vi "CalculateZ.vi"(5 "File Path to Save":path, 7 "EIS File":bool, 8 "Avg I & V":waveform(dbl)[](graph) caption="I & V WFM", 11 "Frequency":dbl format="%.6f") -> (0 "Nyquist Plot":cluster{"Y":dbl[], "Y":dbl[]}[](graph), 1 "ZIm":dbl, 2 "ZRe":dbl, 3 "Current Frequency":dbl format="%.2p", 4 "Ztheta":dbl, 6 "ZMag":dbl)   [LabVIEW 2018]
uses:
  <vilib>/measure/matone.llb/Extract Single Tone Information 1 Chan.vi
  <vilib>/Utility/file.llb/Write To Spreadsheet File (DBL).vi
  <vilib>/measure/NI_MAPro.lvlib
panel:
  out "Avg Voltage":waveform(dbl)(graph)
  out "Avg Current":waveform(dbl)(graph)
  out "Voltage Phase (deg)":dbl format="%.2p"
  out "Voltage Amplitude (V)":dbl format="%.2p"
  out "Voltage Frequency":dbl format="%.2p"
  out "Current Phase (deg)":dbl format="%.2p"
  out "Current Amplitude (A)":dbl format="%.2p"
  # "Inputs"
  # "Outputs"
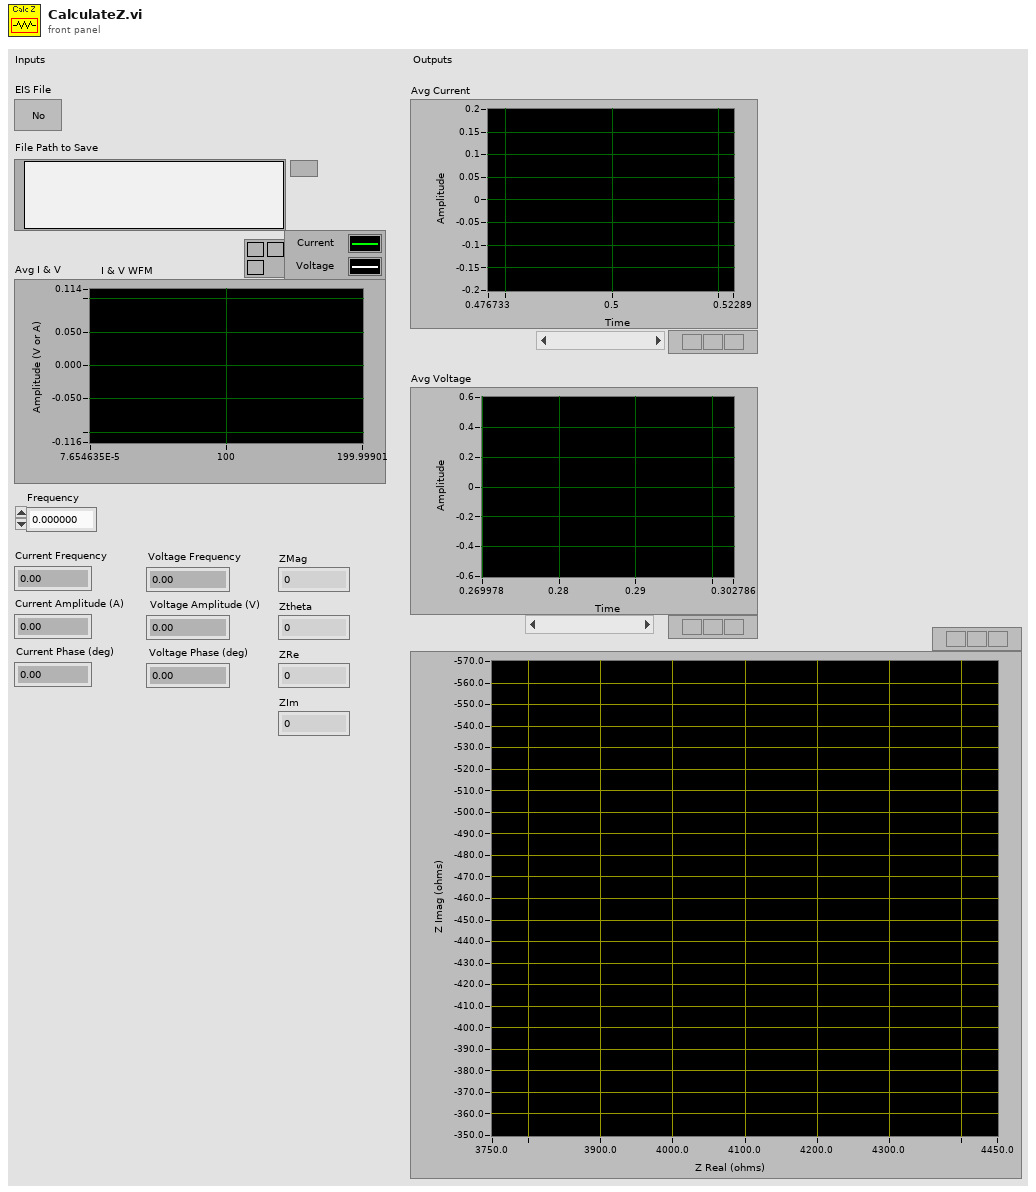
[diagram p1: front panel]
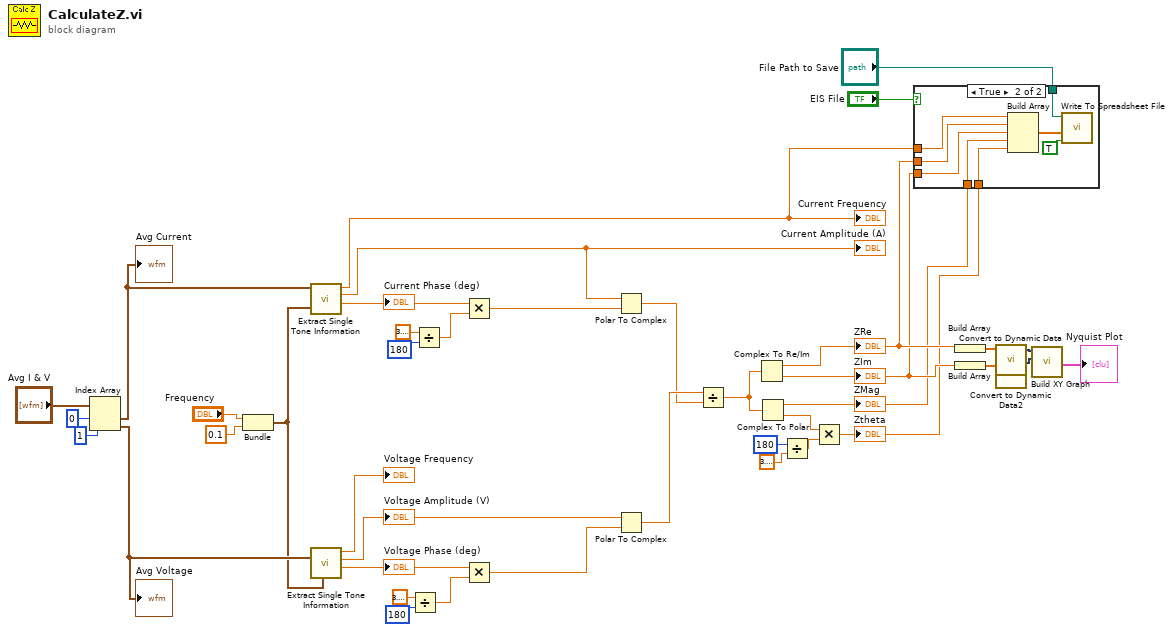
[diagram p0: block diagram]
diagram:
  n1 = Index Array(array="Avg I & V", index #1=0 ("index"), index #2=1 ("index")) -> (element #1=w16:waveform(dbl), element #2=w15:waveform(dbl))
  "Avg Current" <- w16
  "Avg Voltage" <- w15
  n2 = Bundle("Frequency"="Frequency", 0.1) -> (w13:cluster{"Frequency":dbl, dbl})  [unwired: 1 in]
  n3 = call-poly <vilib>:"Extract Single Tone Information.vi"("advanced search"=w13, "time signal in"=w16) -> ("detected phase (deg)"=w29:dbl, "detected amplitude"=w39:dbl, "detected frequency"=w5:dbl)  [unwired: 4 in, 3 out]
  "Current Frequency" <- w5
  "Current Amplitude (A)" <- w39
  "Current Phase (deg)" <- w29
  n4 = call-poly <vilib>:"Extract Single Tone Information.vi"("advanced search"=w13, "time signal in"=w15) -> ("detected phase (deg)"=w34:dbl, "detected amplitude"=w38:dbl, "detected frequency"=→"Voltage Frequency":dbl)  [unwired: 4 in, 3 out]
  "Voltage Amplitude (V)" <- w38
  "Voltage Phase (deg)" <- w34
  n5 = Divide(x=3.141592653589793, y=180) -> (x/y=w35:dbl)
  n6 = Divide(x=3.141592653589793, y=180) -> (x/y=w30:dbl)
  n7 = Multiply(x=w29, y=w30) -> (x*y=w28:dbl)
  n8 = Multiply(x=w34, y=w35) -> (x*y=w33:dbl)
  n9 = Polar To Complex(1:w28, 2:w39) -> (0:w22:cdb)
  n10 = Polar To Complex(1:w33, 2:w38) -> (0:w23:cdb)
  n11 = Divide(x=w23, y=w22) -> (x/y=w21:cdb)
  n12 = Complex To Re/Im(x + iy=w21) -> (x=w4:dbl, y=w3:dbl)
  "ZRe" <- w4
  "ZIm" <- w3
  n13 = Complex To Polar(r * e^(i*theta)=w21) -> (r=w2:dbl, theta=w26:dbl)
  "ZMag" <- w2
  n14 = Divide(x=180, y=3.141592653589793) -> (x/y=w27:dbl)
  n15 = Multiply(x=w26, y=w27) -> (x*y=w1:dbl)
  "Ztheta" <- w1
  n16 = case shown="True" "EIS File" {
    tunnel: w5 -> [_ w46]
    tunnel: w4 -> [_ w45]
    tunnel: w3 -> [_ w44]
    tunnel: "File Path to Save" -> [_ w43]
    tunnel: w2 -> [_ w42]
    tunnel: w1 -> [_ w41]
    frame False {
    }
    frame True {
      n17 = Build Array(w46, w45, w44, w42, w41) -> (w47:dbl[])
      n18 = call-poly <vilib>:"Write To Spreadsheet File.vi"("append to file? (new file:F)"=TRUE, "1D data"=w47, "file path (dialog if empty)"=w43) -> ()  [unwired: 5 in, 1 out]
    }
  }
  n19 = Build Array(w4) -> (w12:dbl[])
  n20 = Build Array(w3) -> (w11:dbl[])
  n21 = call "Convert to Dynamic Data"("Array"=w12) -> ("Dynamic Data Type"=w9:dynamicdata)  [unwired: 3 in]
  n22 = call "Convert to Dynamic Data2"("Array"=w11) -> ("Dynamic Data Type"=w10:dynamicdata)  [unwired: 3 in]
  n23 = call "Build XY Graph"("Y Input"=w10, "X Input"=w9) -> ("XY Graph"=→"Nyquist Plot":cluster{"Y":dbl[], "Y":dbl[]}[])  [unwired: 8 in, 1 out]
